vi "QueuedWriteToDatabase.vi"(8 "error in":errorcluster, 10 "Stop Flag Reference":refnum<vi>, 11 "queue":refnum<queue>) -> (0 "error out":errorcluster)   [LabVIEW 2012]
uses:
  <vilib>/addons/database/Connection.llb/Conn ObjectReference.ctl
  <vilib>/addons/database/NI_Database_API.lvlib
panel:
  out "Database Writing Source":i32
  out "Database Table":string
  out "Database Writing Error":bool
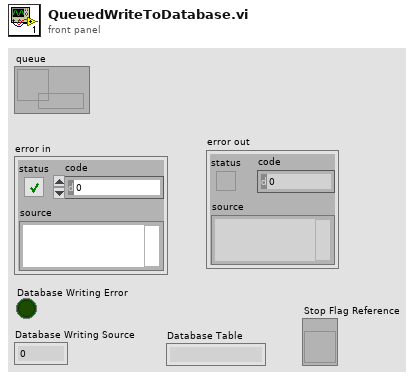
[diagram p1: front panel]
types:
  T1 = cluster{"setup":u8, "session_start_time":u64, "stim_start_time":u64, "time":u64}
  T2 = cluster{"setup":u8, "subject_id":i32, "session_start_time":dbl, "stim_start_time":dbl, "stim_path":path, "exp_type":string}
  T3 = cluster{"setup":u8, "subject_id":i32, "session_start_time":dbl, "stim_start_time":dbl, "time":dbl}
  T4 = cluster{"setup":u8, "subject_id":i32, "session_start_time":dbl, "stim_start_time":dbl, "beh_start_time":dbl, "beh_path":path, "beh_traces_type":string}
  T5 = cluster{"setup":u8, "subject_id":i32, "session_start_time":dbl, "ephys_start_time":dbl, "ephys_path":path, "ephys_task":string}
  T6 = cluster{"setup":u8, "subject_id":u64, "session_start_time":dbl, "channel":u64, "counter":u64, "time":u64}
  T7 = cluster{"setup":u8, "subject_id":i32, "experimenter":string, "session_start_time":dbl, "session_path":path, "session_datetime":timestamp}
  T8 = typedef "NI_Database_API.lvlib/Conn ObjectReference.ctl" = refnum<k1>
  T9 = cluster{cluster{"reference":T8, "table":string, "columns":string[], i32}, "Variant":variant}
  T10 = cluster{"reference":T8, "table":string, "columns":string[], i32}
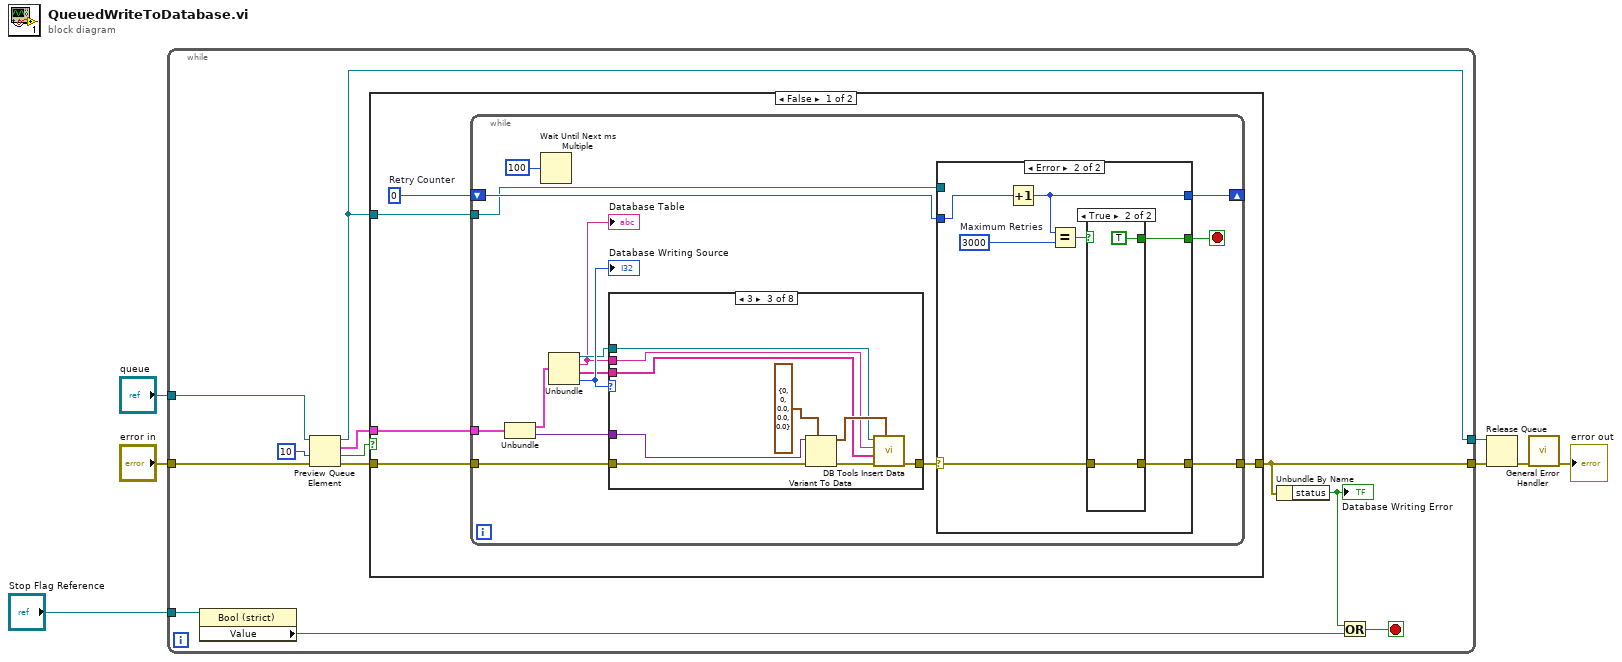
[diagram p0: block diagram]
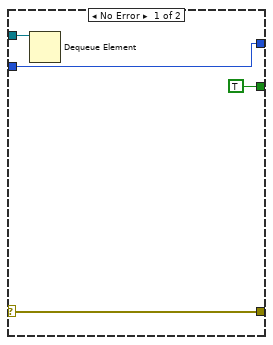
[diagram p2: hidden frame]
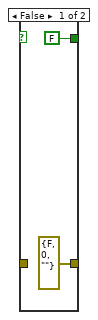
[diagram p3: hidden frame]
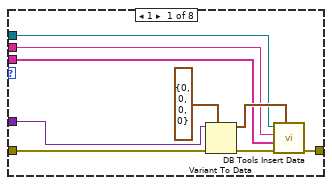
[diagram p4: hidden frame]
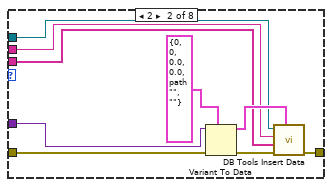
[diagram p5: hidden frame]
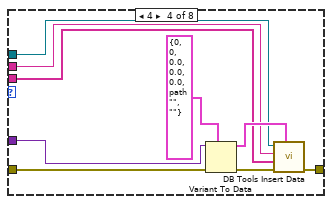
[diagram p6: hidden frame]
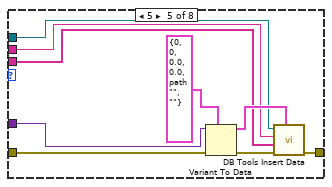
[diagram p7: hidden frame]
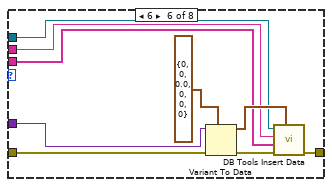
[diagram p8: hidden frame]
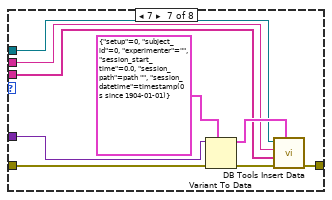
[diagram p9: hidden frame]
diagram:
  n1 = while {
    tunnel: "error in" -> [w12]
    tunnel: [w10] -> w4
    tunnel: [w11] -> w3
    tunnel: "Stop Flag Reference" -> [w14]
    tunnel: "queue" -> [w13]
    stop <- w16 stop-if-true
    n2 = property class="Bool (strict)"(reference=w14) -> ("Value"=w9:bool)  [unwired: 1 in, 2 out]
    n3 = Preview Queue Element(queue=w13, timeout in ms (-1)=10, error in (no error)=w12) -> (queue out=w10:refnum<queue>, element=w15:T9, timed out?=w18:bool, error out=w17:errorcluster)
    n4 = case shown="False" w18 {
      tunnel: w15 -> [w24 _]
      tunnel: w17 -> [w23 w119]
      tunnel: [w21 w119] -> w11
      tunnel: w10 -> [w20 _]
      frame False {
        w22 = 0  # Retry Counter
        n5 = while {
          tunnel: w24 -> [w39]
          tunnel: w23 -> [w35]
          shift-right: [w27] -> _
          shift-left: w22 -> [w29]
          tunnel: [w28] -> w21
          tunnel: w20 -> [w25]
          stop <- w26 stop-if-true
          n6 = Unbundle(w39) -> (w38:T10, "Variant"=w37:variant)
          n7 = Wait Until Next ms Multiple(millisecond multiple=u32 100) -> ()  [unwired: 1 out]
          n8 = Unbundle(w38) -> ("reference"=w34:T8, "table"=w33:string, "columns"=w32:string[], w36:i32)
          "Database Writing Source" <- w36
          "Database Table" <- w33
          n9 = case shown="3" w36 {
            tunnel: w37 -> [w63 w71 w80 w83 w94 w101 w112 _]
            tunnel: w35 -> [w61 w70 w79 w84 w93 w103 w111 w118]
            tunnel: [w55 w64 w73 w85 w92 w102 w110 w118] -> w30
            tunnel: w34 -> [w59 w68 w77 w86 w95 w104 w115 _]
            tunnel: w33 -> [w58 w67 w76 w87 w96 w105 w114 _]
            tunnel: w32 -> [w57 w66 w75 w88 w97 w106 w113 _]
            frame 1 {
              n10 = Variant To Data(error in=w61, type=T1 {"setup"=0, "session_start_time"=0, "stim_start_time"=0, "time"=0} ("output cluster"), Variant=w63) -> (data=w60:T1, error out=w56:errorcluster)
              n11 = call <vilib>:"DB Tools Insert Data.vi"("data"=w60, "error in (no error)"=w56, "columns"=w57, "table"=w58, "connection reference"=w59) -> ("error out"=w55:errorcluster)  [unwired: 5 in, 1 out]
            }
            frame 2 {
              n12 = Variant To Data(error in=w70, type=T2 {"setup"=0, "subject_id"=0, "session_start_time"=0.0, "stim_start_time"=0.0, "stim_path"=path "", "exp_type"=""} ("output cluster"), Variant=w71) -> (data=w69:T2, error out=w65:errorcluster)
              n13 = call <vilib>:"DB Tools Insert Data.vi"("data"=w69, "error in (no error)"=w65, "columns"=w66, "table"=w67, "connection reference"=w68) -> ("error out"=w64:errorcluster)  [unwired: 5 in, 1 out]
            }
            frame 3 {
              n14 = Variant To Data(error in=w79, type=T3 {"setup"=0, "subject_id"=0, "session_start_time"=0.0, "stim_start_time"=0.0, "time"=0.0} ("output cluster"), Variant=w80) -> (data=w78:T3, error out=w74:errorcluster)
              n15 = call <vilib>:"DB Tools Insert Data.vi"("data"=w78, "error in (no error)"=w74, "columns"=w75, "table"=w76, "connection reference"=w77) -> ("error out"=w73:errorcluster)  [unwired: 5 in, 1 out]
            }
            frame 4 {
              n16 = Variant To Data(error in=w84, type=T4 {"setup"=0, "subject_id"=0, "session_start_time"=0.0, "stim_start_time"=0.0, "beh_start_time"=0.0, "beh_path"=path "", "beh_traces_type"=""} ("output cluster"), Variant=w83) -> (data=w89:T4, error out=w90:errorcluster)
              n17 = call <vilib>:"DB Tools Insert Data.vi"("data"=w89, "error in (no error)"=w90, "columns"=w88, "table"=w87, "connection reference"=w86) -> ("error out"=w85:errorcluster)  [unwired: 5 in, 1 out]
            }
            frame 5 {
              n18 = Variant To Data(error in=w93, type=T5 {"setup"=0, "subject_id"=0, "session_start_time"=0.0, "ephys_start_time"=0.0, "ephys_path"=path "", "ephys_task"=""} ("output cluster"), Variant=w94) -> (data=w98:T5, error out=w99:errorcluster)
              n19 = call <vilib>:"DB Tools Insert Data.vi"("data"=w98, "error in (no error)"=w99, "columns"=w97, "table"=w96, "connection reference"=w95) -> ("error out"=w92:errorcluster)  [unwired: 5 in, 1 out]
            }
            frame 6 {
              n20 = Variant To Data(error in=w103, type=T6 {"setup"=0, "subject_id"=0, "session_start_time"=0.0, "channel"=0, "counter"=0, "time"=0} ("output cluster"), Variant=w101) -> (data=w108:T6, error out=w107:errorcluster)
              n21 = call <vilib>:"DB Tools Insert Data.vi"("data"=w108, "error in (no error)"=w107, "columns"=w106, "table"=w105, "connection reference"=w104) -> ("error out"=w102:errorcluster)  [unwired: 5 in, 1 out]
            }
            frame 7 {
              n22 = Variant To Data(error in=w111, type=T7 {"setup"=0, "subject_id"=0, "experimenter"="", "session_start_time"=0.0, "session_path"=path "", "session_datetime"=timestamp(0 s since 1904-01-01)} ("output cluster"), Variant=w112) -> (data=w117:T7, error out=w116:errorcluster)
              n23 = call <vilib>:"DB Tools Insert Data.vi"("data"=w117, "error in (no error)"=w116, "columns"=w113, "table"=w114, "connection reference"=w115) -> ("error out"=w110:errorcluster)  [unwired: 5 in, 1 out]
            }
            frame 0, Default {
            }
          }
          n24 = case shown="Error" w30 {
            selector: w30 -> [w42 w46]
            tunnel: w29 -> [w43 w50]
            tunnel: [w43 w48] -> w27
            tunnel: [w42 w45] -> w28
            tunnel: [TRUE w44] -> w26
            tunnel: w25 -> [w40 _]
            frame No Error {
              n25 = Dequeue Element(queue=w40) -> ()  [unwired: 2 in, 4 out]
            }
            frame Error {
              w47 = 3000  # Maximum Retries
              n26 = Increment(x=w50) -> (x+1=w48:i32)
              n27 = Equal?(x=w48, y=w47) -> (x = y?=w49:bool)
              n28 = case shown="True" w49 {
                tunnel: w46 -> [_ w54]
                tunnel: [errorcluster {"status"=FALSE, "code"=0, "source"=""} ("error IO") w54] -> w45
                tunnel: [FALSE TRUE] -> w44
                frame False {
                }
                frame True {
                }
              }
            }
          }
        }
      }
      frame True {
      }
    }
    n29 = Unbundle By Name(w11) -> ("status"=w8:bool)
    "Database Writing Error" <- w8
    n30 = Or(x=w8, y=w9) -> (x .or. y?=w16:bool)
  }
  n31 = Release Queue(queue=w4, error in (no error)=w3) -> (error out=w5:errorcluster)  [unwired: 1 in, 2 out]
  n32 = call <vilib>:"General Error Handler.vi"("error in (no error)"=w5) -> ("error out"=→"error out":errorcluster)  [unwired: 10 in, 4 out]
